vi "2022-CheesyDriveUpdated.vi"(0 "Throttle":dbl(slide)=-0.0 scale=-1.0..1.0, 1 "Custom MaxSpeedSlow (0.6)":dbl=0.6, 2 "Custom SlowRate (1)":dbl=3.5, 5 "Wheel":dbl(slide) scale=-1.0..1.0, 7 "Cheezy Drive Mode (2)":u16(ring)=3, 9 "CarLikeTurning":bool, 11 "Quickturn":bool, 12 "Custom MaxTurnSlow (0.55)":dbl=0.75, 13 "Custom MaxTurnRateSlow (20)":dbl=20.0) -> (4 "Left PWM":dbl, 6 "Right PWM":dbl)   [LabVIEW 2020]
doc: "Implements CheesyDrive. CheesyDrive means that the turn joystick controls the radius of turning instead of the rate of turning. Also implements QuickStop and QuickTurn."
panel:
  in  "FasterDeaccelerate (3)":dbl=3.0
  in  "EnableHighSensRamp (0.8)":dbl=0.8 format="%#_13g"
  in  "HighSensRamp (7)":dbl=7.0 format="%#_13g"
  in  "ArrayOfSlownesss":T1(array[cluster])=[{"MaxSpeedSlow"=1.0, "SlowRate"=5.0, "MaxTurnSlow"=1.0, "MaxTurnRateSlow"=10.0}, {"MaxSpeedSlow"=0.6, "SlowRate"=4.0, "MaxTurnSlow"=0.8, "MaxTurnRateSlow"=10.0}, {"MaxSpeedSlow"=0.4, "SlowRate"=1.0, "MaxTurnSlow"=0.55, "MaxTurnRateSlow"=10.0}, {"MaxSpeedSlow"=0.6, "SlowRate"=1.0, "MaxTurnSlow"=0.55, "MaxTurnRateSlow"=20.0}] caption="Normal\n\n\n\n\n\n\n\n\n\n\n\n\nSwitch\n\n\n\n\n\n\n\n\n\n\n\nScale\n\n\n\n\n\n\n\n\n\n\n\n\nCustom"
  in  "PointsTurn":cluster{"X":dbl, "Y":dbl}[](array[cluster])=[{"X"=0.0, "Y"=0.0}, {"X"=0.04, "Y"=0.0}, {"X"=0.041, "Y"=0.01}, {"X"=1.0, "Y"=1.0}, {"X"=1.0, "Y"=1.0}]
  in  "PointsQuickTurn":cluster{"X":dbl, "Y":dbl}[](array[cluster])=[{"X"=0.0, "Y"=0.0}, {"X"=0.04, "Y"=0.0}, {"X"=0.041, "Y"=0.2}, {"X"=0.9, "Y"=0.5}, {"X"=1.0, "Y"=1.0}]
  in  "PointsThrottle":cluster{"X":dbl, "Y":dbl}[](array[cluster])=[{"X"=0.0, "Y"=0.0}, {"X"=0.04, "Y"=0.0}, {"X"=0.0251, "Y"=0.15}, {"X"=1.0, "Y"=1.0}]
  in  "QSMult (0.1)":dbl=0.1
  in  "WheelNonLinearity (0.65)":dbl=0.65
  in  "negInertiaScalar (3)":dbl=3.0
  in  "alpha (0.1)":dbl=0.1
  out "Waveform Chart":dbl(graph)
  in  "Sensitivty (1)":dbl=1.0
  # "Enable to enable"
  # "Cheezy Drive Settings"
  # "(for quickstop decay)"
  # "Explanation:\n\"Cheesy Drive\" simply means that\n * the \"turning\" stick controls the curvature of the robot's path rather than\n * its rate of heading change. This helps make the robot more controllable at\n * high speeds. \n\nAlso handles the robot's quick turn functionality - \"quick turn\"\n * overrides constant-curvature turning for turn-in-place maneuvers.\n * Quick Stop applies backwards power to the motors to stop the robot\n * when in quick turn mode, so the robot handles better"
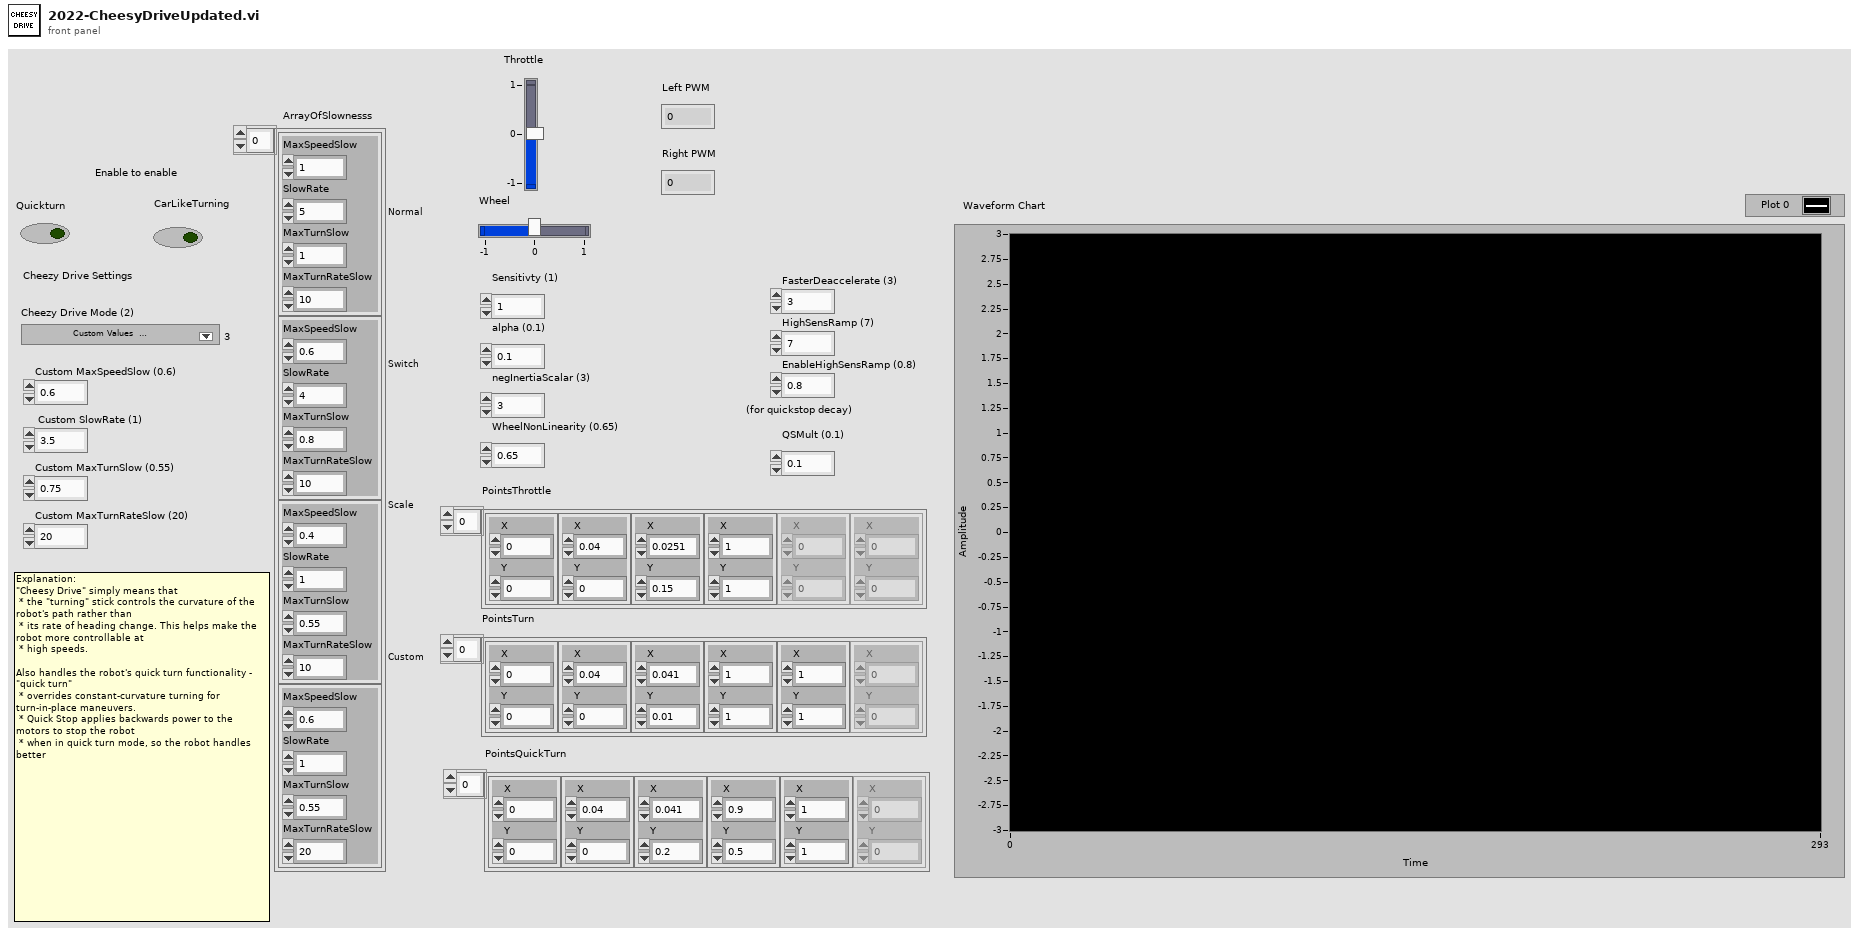
[diagram p1: front panel]
types:
  T1 = cluster{"MaxSpeedSlow":dbl, "SlowRate":dbl, "MaxTurnSlow":dbl, "MaxTurnRateSlow":dbl}[]
  T2 = cluster{"MaxSpeedSlow":dbl, "SlowRate":dbl, "MaxTurnSlow":dbl, "MaxTurnRateSlow":dbl}
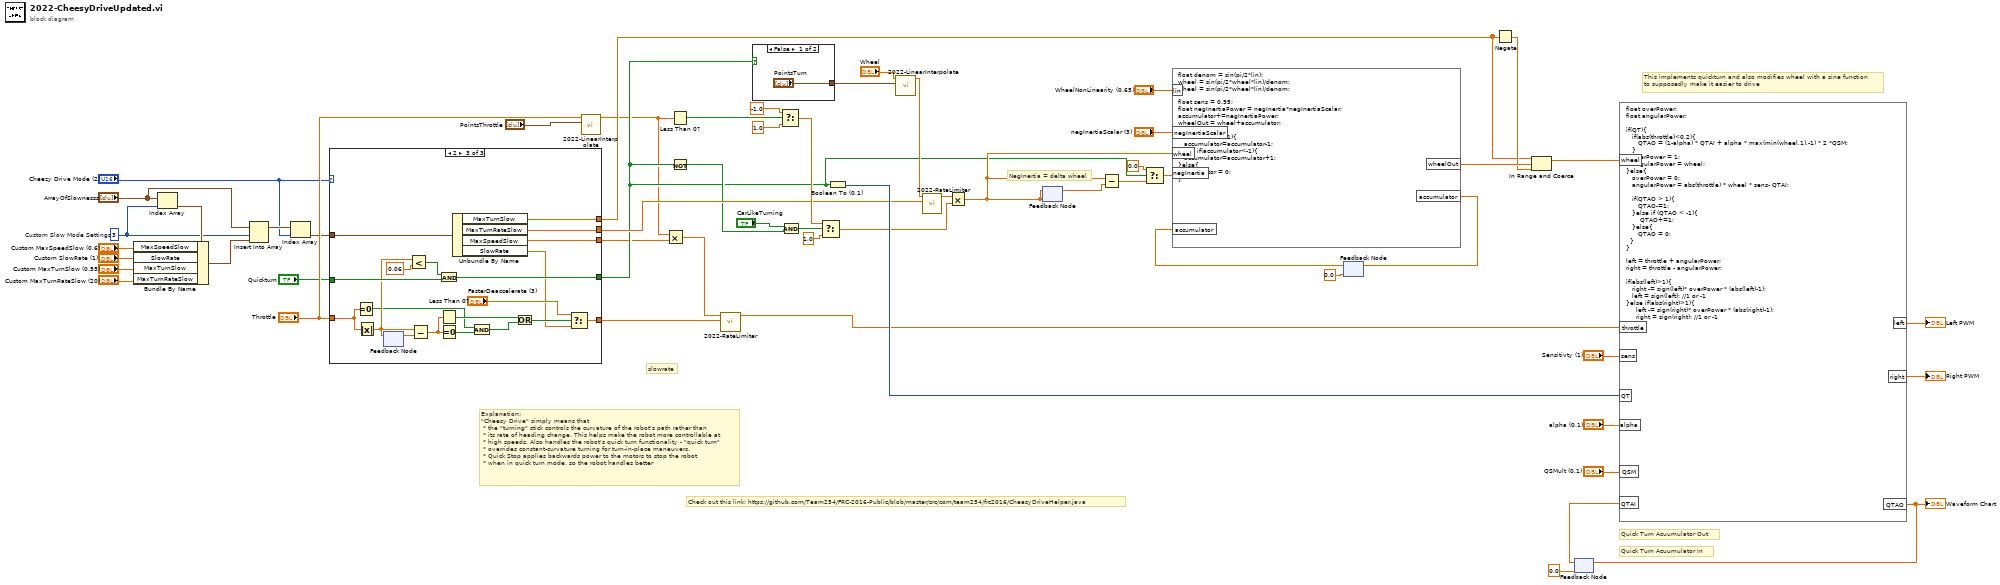
[diagram p0: block diagram]
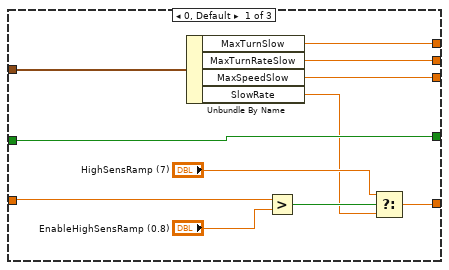
[diagram p2: hidden frame]
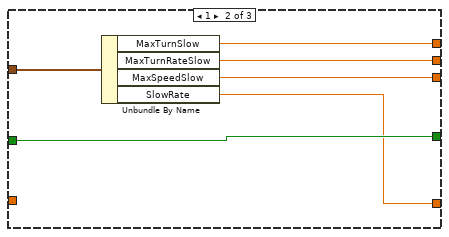
[diagram p3: hidden frame]
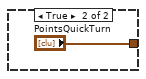
[diagram p4: hidden frame]
diagram:
  w7 = 3  # Custom Slow Mode Settings
  # "slowrate"
  # "This implements quickturn and also modifies wheel with a sine function\nto supposedly make it easier to drive"
  # "NegInertia = delta wheel"
  # "Explanation:\n\"Cheesy Drive\" simply means that\n * the \"turning\" stick controls the curvature of the robot's path rather than\n * its rate of heading change. This helps make the robot more controllable at\n * high speeds. Also handles the robot's quick turn functionality - \"quick turn\"\n * overrides constant-curvature turning for turn-in-place maneuvers.\n * Quick Stop applies backwards power to the motors to stop the robot\n * when in quick turn mode, so the robot handles better"
  # "Quick Turn Acuumulator Out"
  # "Quick Turn Acuumulator In"
  # "Check out this link: https://github.com/Team254/FRC-2016-Public/blob/master/src/com/team254/frc2016/CheesyDriveHelper.java"
  n1 = Index Array(array="ArrayOfSlownesss", index=w7) -> (element=w12:T2)
  n2 = Bundle By Name(cluster=w12, "MaxSpeedSlow"="Custom MaxSpeedSlow (0.6)", "SlowRate"="Custom SlowRate (1)", "MaxTurnSlow"="Custom MaxTurnSlow (0.55)", "MaxTurnRateSlow"="Custom MaxTurnRateSlow (20)") -> (w10:T2)
  n3 = Insert Into Array(array="ArrayOfSlownesss", index=w7, new element=w10) -> (w9:T1)
  n4 = Index Array(array=w9, index="Cheezy Drive Mode (2)") -> (element=w8:T2)
  n5 = case shown="2" "Cheezy Drive Mode (2)" {
    tunnel: [w61 w69 w86] -> w29
    tunnel: [w58 w70 w76] -> w13
    tunnel: [w66 w72 w87] -> w27
    tunnel: [w67 w73 w88] -> w24
    tunnel: "Quickturn" -> [w68 w74 w94]
    tunnel: [w68 w74 w91] -> w16
    tunnel: "Throttle" -> [w65 _ w83]
    tunnel: w8 -> [w60 w71 w77]
    frame 0, Default {
      n6 = Unbundle By Name(w60) -> ("MaxTurnSlow"=w66:dbl, "MaxTurnRateSlow"=w67:dbl, "MaxSpeedSlow"=w58:dbl, "SlowRate"=w59:dbl)
      n7 = Greater?(x=w65, y="EnableHighSensRamp (0.8)") -> (0:w63:bool)
      n8 = Select(t="HighSensRamp (7)", s=w63, f=w59) -> (s? t:f=w61:dbl)
    }
    frame 1 {
      n9 = Unbundle By Name(w71) -> ("MaxTurnSlow"=w72:dbl, "MaxTurnRateSlow"=w73:dbl, "MaxSpeedSlow"=w70:dbl, "SlowRate"=w69:dbl)
    }
    frame 2 {
      n10 = Equal To 0?(x=w83) -> (x = 0?=w82:bool)
      n11 = Absolute Value(x=w83) -> (abs(x)=w89:dbl)
      n12 = feedback-in #1(w89) -> ()
      n13 = feedback #1() -> (w90:dbl)  [unwired: 1 in]
      n14 = Less?(x=w89, y=0.06) -> (x < y?=w93:bool)
      n15 = Subtract(x=w89, y=w90) -> (x-y=w81:dbl)
      n16 = And(x=w93, y=w94) -> (x .and. y?=w91:bool)
      n17 = Less Than 0?(x=w81) -> (x < 0?=w84:bool)
      n18 = Equal To 0?(x=w81) -> (x = 0?=w79:bool)
      n19 = Unbundle By Name(w77) -> ("MaxTurnSlow"=w87:dbl, "MaxTurnRateSlow"=w88:dbl, "MaxSpeedSlow"=w76:dbl, "SlowRate"=w75:dbl)
      n20 = And(x=w82, y=w79) -> (x .and. y?=w80:bool)
      n21 = Or(x=w84, y=w80) -> (x .or. y?=w78:bool)
      n22 = Select(t="FasterDeaccelerate (3)", s=w78, f=w75) -> (s? t:f=w86:dbl)
    }
  }
  n23 = call "2022-LinearInterpolate.vi"("Points"="PointsThrottle", "Value"="Throttle") -> ("Output"=w15:dbl)  [unwired: 9 in]
  n24 = Multiply(x=w15, y=w13) -> (x*y=w14:dbl)
  n25 = Less Than 0?(x=w15) -> (x < 0?=w39:bool)
  n26 = Not(x=w16) -> (.not. x?=w18:bool)
  n27 = call "2022-RateLimiter.vi"("Max dx/dt"=w29, "Input"=w14) -> ("Output"=w51:dbl)  [unwired: 9 in]
  n28 = case shown="False" w16 {
    tunnel: ["PointsTurn" "PointsQuickTurn"] -> w31
    frame False {
    }
    frame True {
    }
  }
  n29 = Select(t=-1.0, s=w39, f=1.0) -> (s? t:f=w35:dbl)
  n30 = And(x="CarLikeTurning", y=w18) -> (x .and. y?=w17:bool)
  n31 = Select(t=w35, s=w17, f=1.0) -> (s? t:f=w33:dbl)
  n32 = Boolean To (0,1)(Boolean=w16) -> (0, 1=w55:i16)
  n33 = call "2022-LinearInterpolate.vi"("Points"=w31, "Value"="Wheel") -> ("Output"=w26:dbl)  [unwired: 9 in]
  n34 = call "2022-RateLimiter.vi"("Max dx/dt"=w24, "Input"=w26) -> ("Output"=w25:dbl)  [unwired: 9 in]
  n35 = Multiply(x=w25, y=w33) -> (x*y=w36:dbl)
  n36 = feedback #2(w36) -> (w48:dbl)
  n37 = feedback-in #2(w36) -> ()
  n38 = Subtract(x=w36, y=w48) -> (x-y=w22:dbl)
  n39 = Select(t=0.0, s=w16, f=w22) -> (s? t:f=w23:dbl)
  n40 = feedback #3(0.0 ("Wheel")) -> (w47:dbl)
  n41 = formula code="float denom = sin(pi/2*lin);\nwheel = sin(pi/2*wheel*lin)/denom;\nwheel = sin(pi/2*wheel*lin)/denom;\n\nfloat sens = 0.95;\nfloat negInertiaPower = negInertia*negInertiaScalar;\naccumulator+=negInertiaPower;\nwheelOut = wheel+accumulator;\n\nif(accumulator>1){\n   accumulator=accumulator-1;\n}else if(accumulator<-1){\n   accumulator=accumulator+1;\n}else{\naccumulator = 0;\n}"("wheel"=w36, "negInertia"=w23, "accumulator"=w47, "negInertiaScalar"="negInertiaScalar (3)", "lin"="WheelNonLinearity (0.65)") -> ("accumulator"=w45:dbl, "wheelOut"=w41:dbl)
  n42 = feedback-in #3(w45) -> ()
  n43 = Negate(x=w27) -> (-x=w28:dbl)
  n44 = In Range and Coerce(upper limit=w27, x=w41, lower limit=w28) -> (coerced(x)=w42:dbl)  [unwired: 1 out]
  n45 = feedback #4(0.0 ("QTAccumulatorO")) -> (w53:dbl)
  n46 = formula code="float overPower;\nfloat angularPower;\n\nif(QT){\n   if(abs(throttle)<0.2){\n      QTAO = (1-alpha) * QTAI + alpha * max(min(wheel,1),-1) * 2 *QSM;\n   }\n   overPower = 1;\n   angularPower = wheel;\n}else{\n   overPower = 0;\n   angularPower = abs(throttle) * wheel * sens- QTAI;\n\n   if(QTAO > 1){\n      QTAO-=1;\n   }else if (QTAO < -1){\n       QTAO+=1;\n   }else{\n      QTAO = 0;\n  }\n}\n\nleft = throttle + angularPower;\nright = throttle - angularPower;\n\nif(abs(left)>1){\n   right -= sign(left)* overPower * (abs(left)-1);\n   left = sign(left); //1 or -1\n}else if(abs(right)>1){\n     left -= sign(right)* overPower * (abs(right)-1);\n     right = sign(right); //1 or -1 \n}"("wheel"=w42, "throttle"=w51, "sens"="Sensitivty (1)", "QT"=w55, "alpha"="alpha (0.1)", "QTAI"=w53, "QSM"="QSMult (0.1)") -> ("left"=→"Left PWM":dbl, "right"=→"Right PWM":dbl, "QTAO"=w56:dbl)
  "Waveform Chart" <- w56
  n47 = feedback-in #4(w56) -> ()
